vi "main_ok.vi"() -> ()   [LabVIEW 2013]
panel:
  in  "?":bool=TRUE
  out "Waveform Chart":dbl(graph)=-32.0
  in  "stop":bool
  out "DDP":string="-32\r\n"
  out "Porta livre?":bool=TRUE
  in  "baud rate (9600)":u32=115200
  in  "VISA Refnum in":refnum<visa-resource-name>="COM3"
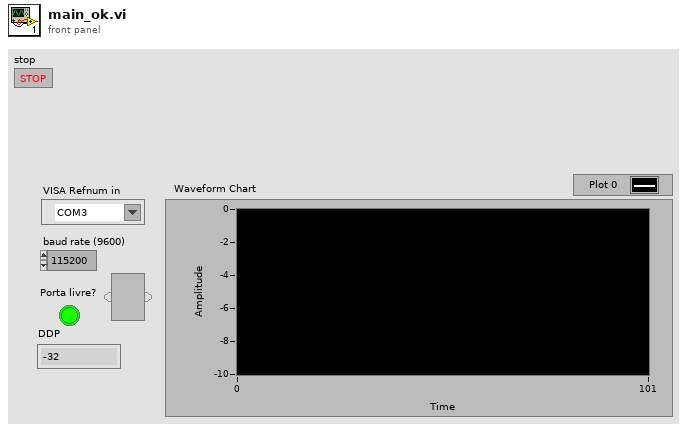
[diagram p1: front panel]
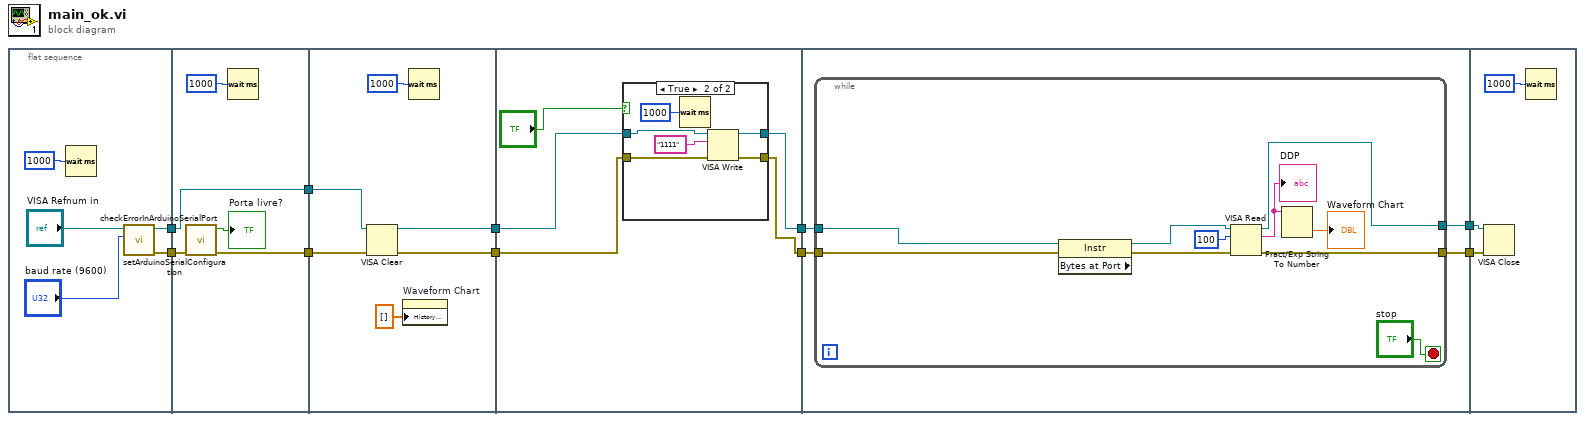
[diagram p0: block diagram]
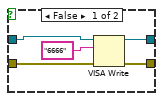
[diagram p2: hidden frame]
diagram:
  n1 = flat-sequence {
    tunnel: [w15] -> w8
    tunnel: [w14] -> w7
    tunnel: [w17] -> w10
    tunnel: [w20] -> w9
    tunnel: w8 -> [w20]
    tunnel: w7 -> [w18]
    tunnel: w10 -> [w26]
    tunnel: w9 -> [w25]
    tunnel: [w23] -> w2
    tunnel: [w22] -> w4
    tunnel: w4 -> [w28]
    tunnel: [w30] -> w3
    tunnel: w2 -> [w31]
    tunnel: [w29] -> w1
    tunnel: [w46] -> w6
    tunnel: [w45] -> w5
    tunnel: w3 -> [w43]
    tunnel: w1 -> [w44]
    tunnel: w6 -> [w58]
    tunnel: w5 -> [w57]
    frame #0 {
      n2 = Wait (ms)(milliseconds to wait=u32 1000) -> ()  [unwired: 1 out]
      n3 = call "setArduinoSerialConfiguration.vi"("baud rate (9600)"="baud rate (9600)", "VISA Refnum in"="VISA Refnum in") -> ("error out"=w14:errorcluster, "VISA Refnum out"=w15:refnum<visa-resource-name>)  [unwired: 8 in]
    }
    frame #1 {
      n4 = call "checkErrorInArduinoSerialPort.vi"("error in (no error)"=w18) -> ("error out"=w17:errorcluster, "Porta livre?"=→"Porta livre?":bool)  [unwired: 9 in]
      n5 = Wait (ms)(milliseconds to wait=u32 1000) -> ()  [unwired: 1 out]
    }
    frame #2 {
      n6 = VISA Clear(VISA resource name=w25, error in (no error)=w26) -> (VISA resource name out=w23:refnum<visa-resource-name>, error out=w22:errorcluster)
      n7 = property on="Waveform Chart" class="WFChart (strict)"("History Data"=dbl[] []) -> ()  [unwired: 2 in, 2 out]
      n8 = Wait (ms)(milliseconds to wait=u32 1000) -> ()  [unwired: 1 out]
    }
    frame #3 {
      n9 = case shown="True" "?" {
        tunnel: w31 -> [w36 w42]
        tunnel: w28 -> [w34 w40]
        tunnel: [w35 w41] -> w29
        tunnel: [w33 w39] -> w30
        frame False {
          n10 = VISA Write(VISA resource name=w36, write buffer="6666", error in (no error)=w34) -> (VISA resource name out=w35:refnum<visa-resource-name>, error out=w33:errorcluster)  [unwired: 1 out]
        }
        frame True {
          n11 = Wait (ms)(milliseconds to wait=u32 1000) -> ()  [unwired: 1 out]
          n12 = VISA Write(VISA resource name=w42, write buffer="1111", error in (no error)=w40) -> (VISA resource name out=w41:refnum<visa-resource-name>, error out=w39:errorcluster)  [unwired: 1 out]
        }
      }
    }
    frame #4 {
      n13 = while {
        tunnel: [w53] -> w46
        tunnel: [w55] -> w45
        tunnel: w44 -> [w51]
        tunnel: w43 -> [w50]
        stop <- "stop" stop-if-true
        n14 = property class="Instr" props=["Bytes at Port"](reference=w51, error in=w50) -> (reference out=w56:refnum<visa-resource-name>, error out=w54:errorcluster)  [unwired: 1 out]
        n15 = VISA Read(VISA resource name=w56, byte count=u32 100, error in (no error)=w54) -> (VISA resource name out=w55:refnum<visa-resource-name>, read buffer=w49:string, error out=w53:errorcluster)  [unwired: 1 out]
        "DDP" <- w49
        n16 = Fract/Exp String To Number(string=w49) -> (number=→"Waveform Chart":dbl)  [unwired: 3 in, 1 out]
      }
    }
    frame #5 {
      n17 = VISA Close(VISA resource name=w57, error in (no error)=w58) -> ()  [unwired: 1 out]
      n18 = Wait (ms)(milliseconds to wait=u32 1000) -> ()  [unwired: 1 out]
    }
  }
